vi "Simulator DMM Measure.vi"(7 "DMM Stimulus":T1, 8 "error in (no error)":errorcluster) -> (0 "error out":errorcluster {"code" format="%.0x"}, 2 "DMM Measurement":T2 caption="This reading is allways in the base units\ni.e. V, A, Ohms, Hz, Sec, etc." format="%#_10f")   [LabVIEW 2011]
uses:
  DMM Measurement.ctl
  tests/DC Attenuation/TypeDefs/DCA Stimulus Parameters.ctl
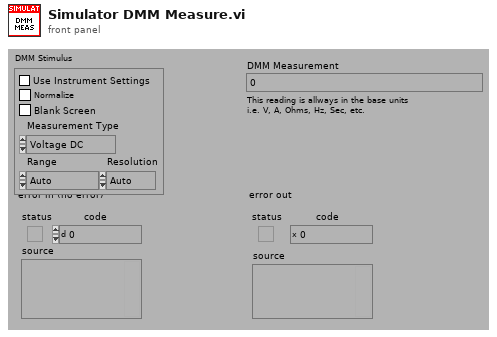
[diagram p1: front panel]
types:
  T1 = typedef "DCA Stimulus Parameters.ctl" = cluster{"Use Instrument":bool, "Normalize":bool, "Blank Screen":bool, "Measurement Type":enum16{"Voltage DC", "Voltage DC Ratio", "Voltage AC", "Current DC", "Current AC", "Resistance", "Fresistance", "Frequency", "Period", "Continuity", "Diode"}, "Range":enum16{"Auto", "Minimum", "Maximum", "100", "1,000", "10,000", "100,000", "1,000,000", "10,000,000", "100,000,000"}, "Resolution":enum16{"Auto", "4 1/2", "5 1/2", "6 1/2"}}
  T2 = typedef "DMM Measurement.ctl" = dbl
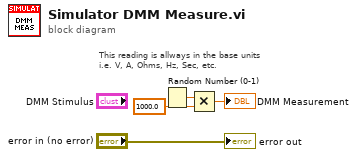
[diagram p0: block diagram]
diagram:
  # "This reading is allways in the base units\ni.e. V, A, Ohms, Hz, Sec, etc."
  n1 = Random Number (0-1)() -> (number: 0 to 1=w3:dbl)
  n2 = Multiply(x=w3, y=1000.0) -> (x*y=→"DMM Measurement":dbl)
  "error out" <- "error in (no error)"
